vi "P3.4.vi"() -> ()   [LabVIEW 2020]
panel:
  in  "stop":bool
  out "Modulo":dbl[](graph)
  out "X 2":dbl[](array[numeric])
  out "X":dbl[](array[numeric])
  out "FFT {X}":cdb[](array[numeric])
  in  "FFT size":i32=-1
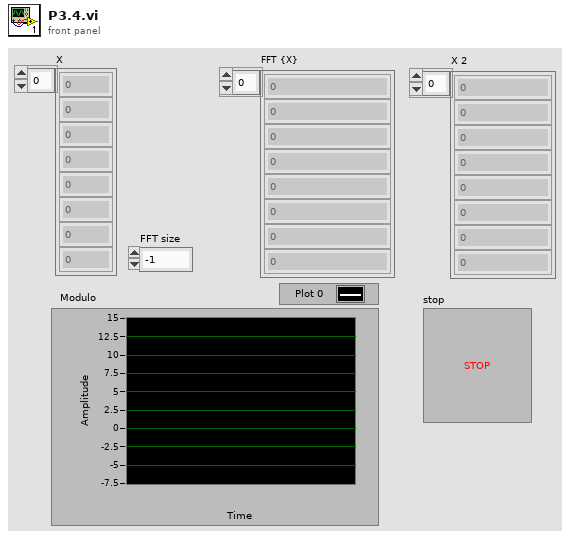
[diagram p1: front panel]
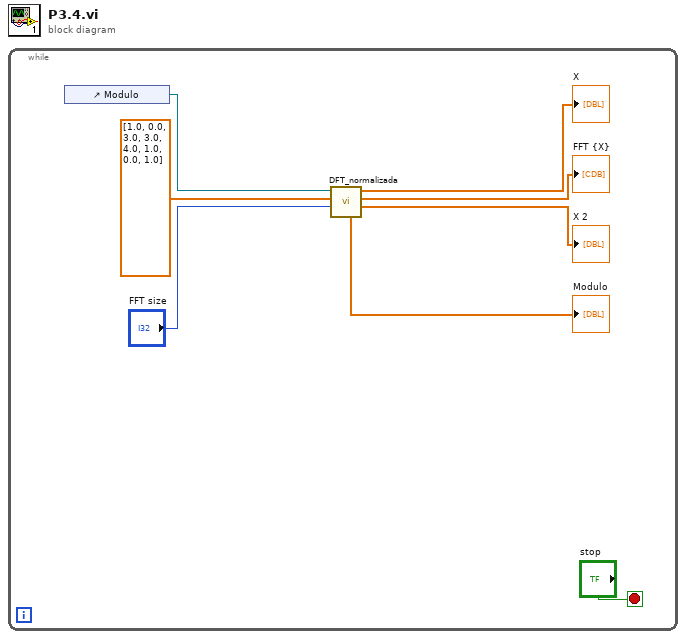
[diagram p0: block diagram]
diagram:
  n1 = while {
    stop <- "stop" stop-if-true
    n2 = control-ref of="Modulo"() -> (w4:refnum<vi>)
    n3 = call "DFT_normalizada.vi"("FFT size"="FFT size", "Length"=dbl[] [1.0, 0.0, 3.0, 3.0, 4.0, 1.0, 0.0, 1.0] ("X"), "WaveformGraph in"=w4) -> ("IFFT( X)"=→"X 2":dbl[], "FFT {X}"=→"FFT {X}":cdb[], "X[n]"=→"X":dbl[], "Array"=→"Modulo":cdb[])  [unwired: 5 in]
  }
